vi "Easy XML Editor Menu.vi"(8 "error in (no error)":errorcluster, 11 "Menu Refnum In":refnum<k9>) -> (0 "error out":errorcluster, 3 "Menu Refnum Out":refnum<k9>)   [LabVIEW 2026, in "VILab.lvlib"]
uses:
  VILab.lvlib
  <vilib>/Utility/miscctls.llb/LVMenuShortCut.ctl
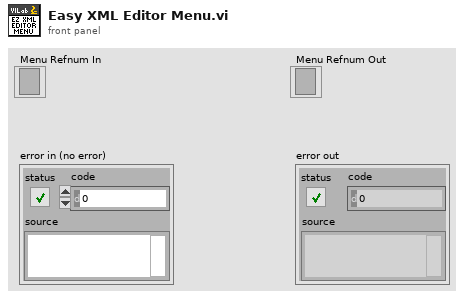
[diagram p1: front panel]
types:
  T1 = typedef "LVMenuShortCut.ctl" = cluster{"Include Shift Key?":bool, "Include Ctrl Key?":bool, "Shortcut Key":string}
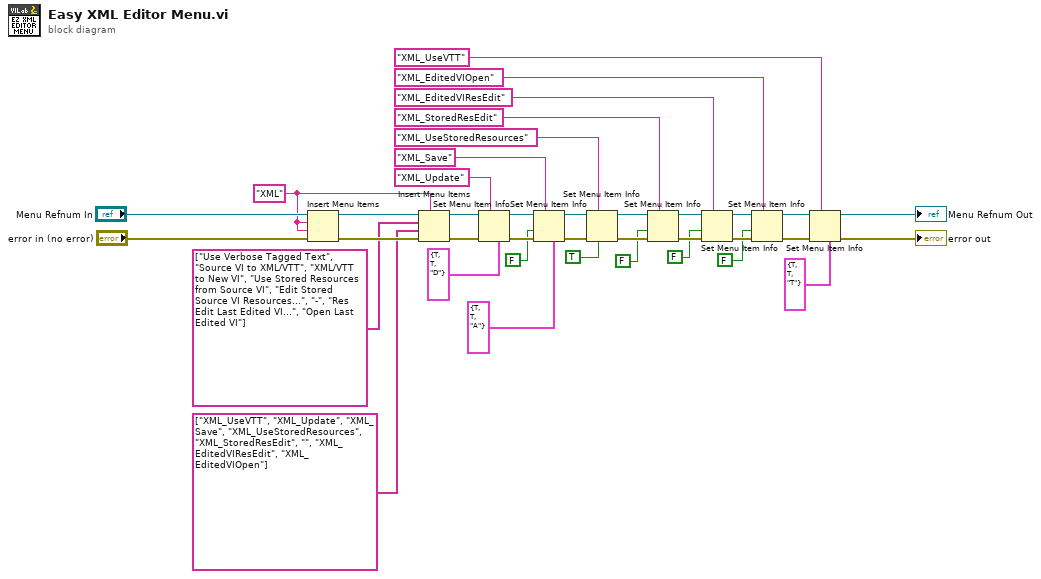
[diagram p0: block diagram]
diagram:
  w22 = "XML"
  n1 = Insert Menu Items(6:"error in (no error)", 7:w22, 8:w22, 9:"Menu Refnum In") -> (0:w33:errorcluster, 3:w34:refnum<k9>)  [unwired: 2 in, 1 out]
  n2 = Insert Menu Items(5:w22, 6:w33, 7:string[] ["XML_UseVTT", "XML_Update", "XML_Save", "XML_UseStoredResources", "XML_StoredResEdit", "", "XML_EditedVIResEdit", "XML_EditedVIOpen"] ("item tags"), 8:string[] ["Use Verbose Tagged Text", "Source VI to XML/VTT", "XML/VTT to New VI", "Use Stored Resources from Source VI", "Edit Stored Source VI Resources...", "-", "Res Edit Last Edited VI...", "Open Last Edited VI"] ("item names"), 9:w34) -> (0:w29:errorcluster, 3:w30:refnum<k9>)  [unwired: 1 in, 1 out]
  n3 = Set Menu Item Info(4:T1 {"Include Shift Key?"=TRUE, "Include Ctrl Key?"=TRUE, "Shortcut Key"="D"} ("short cut"), 7:"XML_Update", 8:w29, 11:w30) -> (0:w27:errorcluster, 3:w26:refnum<k9>)  [unwired: 3 in]
  n4 = Set Menu Item Info(4:T1 {"Include Shift Key?"=TRUE, "Include Ctrl Key?"=TRUE, "Shortcut Key"="A"} ("short cut"), 7:"XML_Save", 8:w27, 9:FALSE, 11:w26) -> (0:w21:errorcluster, 3:w20:refnum<k9>)  [unwired: 2 in]
  n5 = Set Menu Item Info(6:TRUE, 7:"XML_UseStoredResources" ("item tag"), 8:w21, 11:w20) -> (0:w17:errorcluster, 3:w16:refnum<k9>)  [unwired: 3 in]
  n6 = Set Menu Item Info(7:"XML_StoredResEdit", 8:w17, 9:FALSE, 11:w16) -> (0:w14:errorcluster, 3:w13:refnum<k9>)  [unwired: 3 in]
  n7 = Set Menu Item Info(7:"XML_EditedVIResEdit", 8:w14, 9:FALSE, 11:w13) -> (0:w8:errorcluster, 3:w7:refnum<k9>)  [unwired: 3 in]
  n8 = Set Menu Item Info(7:"XML_EditedVIOpen" ("item tag"), 8:w8, 9:FALSE, 11:w7) -> (0:w3:errorcluster, 3:w4:refnum<k9>)  [unwired: 3 in]
  n9 = Set Menu Item Info(4:T1 {"Include Shift Key?"=TRUE, "Include Ctrl Key?"=TRUE, "Shortcut Key"="T"} ("short cut"), 7:"XML_UseVTT" ("item tag"), 8:w3, 11:w4) -> (0:→"error out":errorcluster, 3:→"Menu Refnum Out":refnum<k9>)  [unwired: 3 in]
